vi "hextodate.vi"(0 "object in":refnum<class "interface.lvclass">, 1 "数组":u16[](array[numeric]) format="%04xH", 5 "error in (no error)":errorcluster) -> (14 "object out":refnum<class "interface.lvclass">, 15 "DATE":timestamp[](array[timestamp]), 19 "error out":errorcluster)   [LabVIEW 2016, in "interface.lvclass"]
uses:
  interface.lvclass
  <vilib>/Utility/miscctls.llb/LVDateTimeRec.ctl
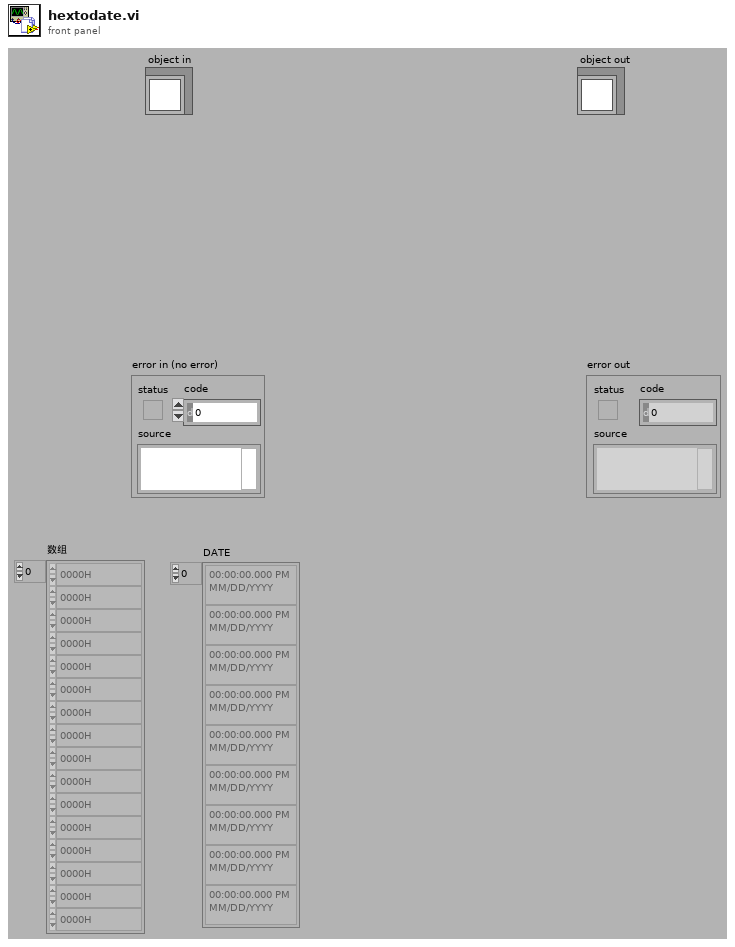
[diagram p1: front panel]
types:
  T1 = typedef "LVDateTimeRec.ctl" = cluster{"fractional second":dbl, "second":i32, "minute":i32, "hour":i32, "day of month":i32, "month":i32, "year":i32, "day of week":i32, "day of year":i32, "DST":i32}
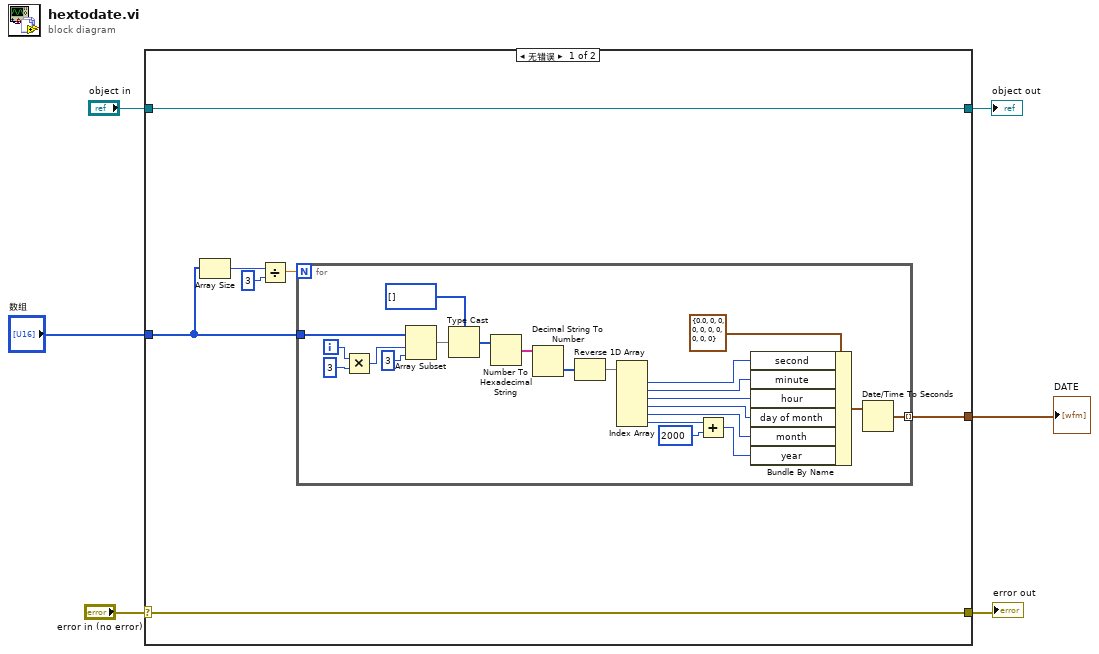
[diagram p0: block diagram]
diagram:
  n1 = case shown="无错误" "error in (no error)" {
    selector: "error in (no error)" -> [w13 w37]
    tunnel: [w13 w37] -> w5
    tunnel: [w12 w36] -> w3
    tunnel: "object in" -> [w12 w36]
    tunnel: "数组" -> [w8 _]
    tunnel: [w7 _] -> w1
    frame No Error {
      n2 = Array Size(array=w8) -> (size(s)=w11:i32)
      n3 = Divide(x=w11, y=3) -> (x/y=w9:dbl)
      n4 = for {
        N: w9 -> [_]
        tunnel: w8 -> [w35]
        tunnel: [w18] -> w7 mode=indexing
        i -> [w34]
        n5 = Multiply(x=w34, y=3) -> (x*y=w31:i32)
        n6 = Array Subset(array=w35, index=w31, length=3 ("索引")) -> (w30:u16[])
        n7 = Type Cast(type=u8[] [], x=w30) -> (*(type *) &x=w16:u8[])
        n8 = Number To Hexadecimal String(2:w16) -> (0:w15:string[])  [unwired: 1 in]
        n9 = Decimal String To Number(string=w15) -> (number=w14:i32[])  [unwired: 2 in, 1 out]
        n10 = Reverse 1D Array(array=w14) -> (reversed array=w17:i32[])
        n11 = Index Array(array=w17) -> (element #1=w27:i32, element #2=w26:i32, element #3=w25:i32, element #4=w24:i32, element #5=w23:i32, element #6=w22:i32)  [unwired: 6 in]
        n12 = Add(x=w22, y=2000) -> (x+y=w20:i32)
        n13 = Bundle By Name(cluster=T1 {"fractional second"=0.0, "second"=0, "minute"=0, "hour"=0, "day of month"=0, "month"=0, "year"=0, "day of week"=0, "day of year"=0, "DST"=0} ("日期时间记录"), "second"=w27, "minute"=w26, "hour"=w25, "day of month"=w24, "month"=w23, "year"=w20) -> (w19:T1)
        n14 = Date/Time To Seconds(2:w19) -> (0:w18:timestamp)  [unwired: 1 in]
      }
    }
    frame Error {
    }
  }
  "error out" <- w5
  "object out" <- w3
  "DATE" <- w1
